vi "Read File Size.vi"(8 "Error In":errorcluster) -> (0 "Error Out":errorcluster)   [LabVIEW 2018, in "Tests.lvlib" / "SFTP Attributes.lvlib"]
uses:
  SFTP Attributes.lvlib
  src/Toolkit/SFTP Attributes/SFTP Attributes.lvclass/SFTP Attributes.ctl
  src/Toolkit/SSH/SSH.lvclass/SSH.ctl
  src/Toolkit/SSH/Utility/Read Shared Library.vi
  src/Toolkit/Support/Check Status.vi
  <vilib>/addons/_JKI Toolkits/Caraya/classes/Test/Test.lvclass
  <vilib>/addons/_JKI Toolkits/Caraya/classes/Assert/Assert.lvclass
  src/Toolkit/SFTP Attributes/SFTP Attributes.lvclass
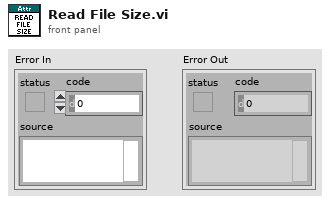
[diagram p1: front panel]
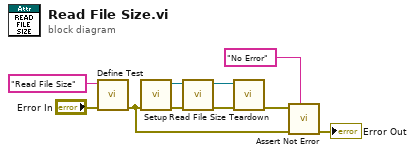
[diagram p0: block diagram]
diagram:
  n1 = call <vilib>:"Define Test.vi"("error in (no error)"="Error In", "Label (VI Title)"="Read File Size") -> ("error out"=w6:errorcluster)  [unwired: 9 in]
  n2 = call "Setup.vi"("Error In"=w6) -> ("Error Out"=w5:errorcluster, "SFTP Attributes"=w4:refnum<class "SFTP Attributes.lvclass">)  [unwired: 9 in]
  n3 = call "Read File Size.vi"("Error In"=w5, "SFTP Attributes In"=w4) -> ("Error Out"=w2:errorcluster, "SFTP Attributes Out"=w3:refnum<class "SFTP Attributes.lvclass">)  [unwired: 7 in, 1 out]
  n4 = call "Teardown.vi"("Error In"=w2, "SFTP Attributes"=w3) -> ("Error Out"=w1:errorcluster)  [unwired: 9 in]
  n5 = call <vilib>:"Assert Not Error.vi"("Label"="No Error", "error in (no error)"=w6, "Not Error?"=w1) -> ("error out"=→"Error Out":errorcluster)  [unwired: 8 in]
